vi "Allgemein_Search_Key.vi"(9 "Teil-Array":string[](array[string]), 10 "length (Eingang)":i32, 11 "index of Options":i32) -> (3 "length (Ausgang)":i32)   [LabVIEW 2020, in "System Einstellungen V2.lvlib"]
uses:
  System Einstellungen V2.lvlib
  <vilib>/regexp/Match Regular Expression.xnode
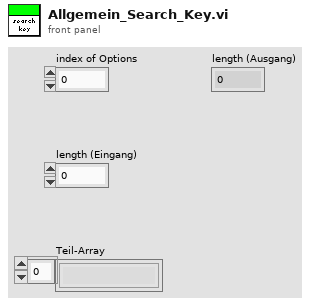
[diagram p1: front panel]
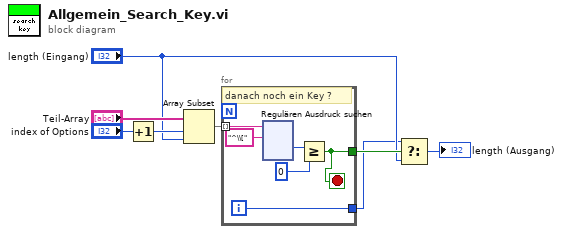
[diagram p0: block diagram]
diagram:
  n1 = Increment(x="index of Options") -> (x+1=w8:i32)
  n2 = Array Subset(array="Teil-Array", index=w8, length="length (Eingang)") -> (w5:string[])
  n3 = for {
    tunnel: w5 -> [w14] mode=indexing
    tunnel: [w10] -> w6
    tunnel: [w9] -> w1
    i -> [w9]
    stop <- w10 stop-if-true
    # "danach noch ein Key ?"
    n4 = xnode "Regulären Ausdruck suchen"("Eingangs-String"=w14, "Regulärer Ausdruck"="^\\[") -> ("Offset nach Übereinstimmung"=w12:i32)  [unwired: 4 in, 4 out]
    n5 = Greater Or Equal?(x=w12, y=0) -> (x >= y?=w10:bool)
  }
  n6 = Select(t=w1, s=w6, f="length (Eingang)") -> (s? t:f=→"length (Ausgang)":i32)
